vi "Check For and Apply Collisions.vi"(1 "Simulation Objects in":refnum<class "SimulationObject.lvclass">[](array[class]), 2 "Collision Grid":refnum<class "CollisionGrid.lvclass">) -> (0 "Simulation Objects out":refnum<class "SimulationObject.lvclass">[](array[class]))   [LabVIEW 2022 SP3, in "CollisionGrid.lvclass"]
uses:
  CollisionGrid.lvclass
  SimulationObject/SimulationObject.lvclass
  CollisionGrid.lvclass/CollisionGrid.ctl
  Collider/Collider.lvclass
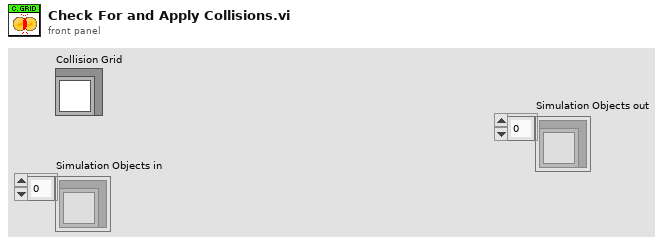
[diagram p1: front panel]
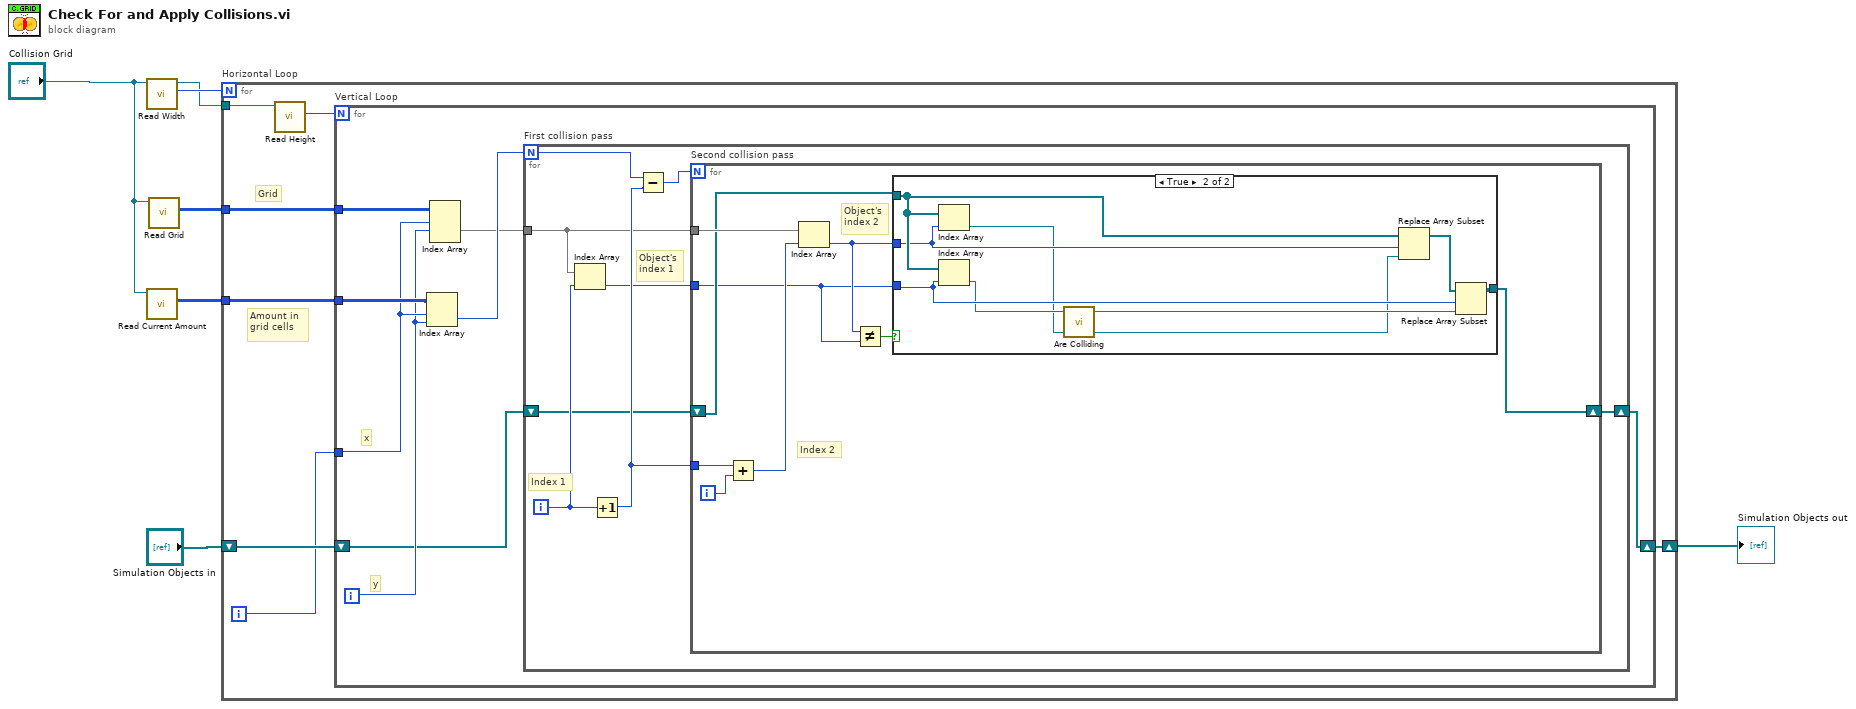
[diagram p0: block diagram]
diagram:
  n1 = call "Read Width.vi"("CollisionGrid in"="Collision Grid") -> ("Width"=w7:i8, "CollisionGrid out"=w6:refnum<class "CollisionGrid.lvclass">)  [unwired: 8 in, 1 out]
  n2 = call "Read Current Amount.vi"("CollisionGrid in"="Collision Grid") -> ("Current Amount"=w1:i16[][])  [unwired: 8 in, 2 out]
  n3 = call "Read Grid.vi"("CollisionGrid in"="Collision Grid") -> ("Grid"=w2:i16[][][])  [unwired: 8 in, 2 out]
  n4 = for "Horizontal Loop" {
    N: w7 -> [_]
    tunnel: w6 -> [w13]
    shift-right: [w11] -> w4
    shift-left: "Simulation Objects in" -> [w12]
    tunnel: w2 -> [w10]
    tunnel: w1 -> [w9]
    i -> [w8]
    # "Amount in grid cells"
    # "Grid"
    n5 = call "Read Height.vi"("CollisionGrid in"=w13) -> ("Height"=w14:i8)  [unwired: 8 in, 2 out]
    n6 = for "Vertical Loop" {
      N: w14 -> [_]
      shift-right: [w15] -> w11
      shift-left: w12 -> [w16]
      tunnel: w10 -> [w22]
      tunnel: w9 -> [w21]
      tunnel: w8 -> [w20]
      i -> [w19]
      # "y"
      # "x"
      n7 = Index Array(array=w21, index (row)=w20, index (col)=w19) -> (element=w18:i16)
      n8 = Index Array(array=w22, index (dim 0)=w20, index (dim 1)=w19) -> (element=w17:i16[])  [unwired: 1 in]
      n9 = for "First collision pass" {
        N: w18 -> [w29]
        tunnel: w17 -> [w27]
        shift-right: [w23] -> w15
        shift-left: w16 -> [w25]
        i -> [w26]
        # "Object's\nindex 1"
        # "Index 1"
        n10 = Index Array(array=w27, index=w26) -> (element=w24:i16)
        n11 = Increment(x=w26) -> (x+1=w28:i32)
        n12 = Subtract(x=w29, y=w28) -> (x-y=w30:i32)
        n13 = for "Second collision pass" {
          N: w30 -> [_]
          tunnel: w27 -> [w37]
          tunnel: w28 -> [w38]
          tunnel: w24 -> [w32]
          shift-right: [w34] -> w23
          shift-left: w25 -> [w35]
          i -> [w39]
          # "Object's\nindex 2"
          # "Index 2"
          n14 = Add(x=w38, y=w39) -> (x+y=w36:i32)
          n15 = Index Array(array=w37, index=w36) -> (element=w33:i16)
          n16 = Not Equal?(x=w33, y=w32) -> (x != y?=w31:bool)
          n17 = case shown="True" w31 {
            tunnel: w35 -> [w40 w48]
            tunnel: w33 -> [_ w47]
            tunnel: w32 -> [_ w46]
            tunnel: [w40 w45] -> w34
            frame False {
            }
            frame True {
              n18 = Index Array(array=w48, index=w47) -> (element=w43:refnum<class "SimulationObject.lvclass">)
              n19 = Index Array(array=w48, index=w46) -> (element=w44:refnum<class "SimulationObject.lvclass">)
              n20 = call "Are Colliding.vi"("Self Object in"=w43, "Other Object in"=w44) -> ("Other Object out"=w41:refnum<class "SimulationObject.lvclass">, "Self Object out"=w42:refnum<class "SimulationObject.lvclass">)  [unwired: 1 in, 1 out]
              n21 = Replace Array Subset(array=w48, new element=w41, index=w47) -> (w49:refnum<class "SimulationObject.lvclass">[])
              n22 = Replace Array Subset(array=w49, new element=w42, index=w46) -> (w45:refnum<class "SimulationObject.lvclass">[])
            }
          }
        }
      }
    }
  }
  "Simulation Objects out" <- w4
